vi "JsonFile Load.vi"(8 "error in (no error)":errorcluster, 11 "Path":path) -> (0 "error out":errorcluster, 3 "Json":string)   [LabVIEW 2019, in "lv-apt-json-file.lvlib"]
uses:
  lv-apt-json-file.lvlib
  <vilib>/JDP Science/JSONtext/JSONtext.lvlib
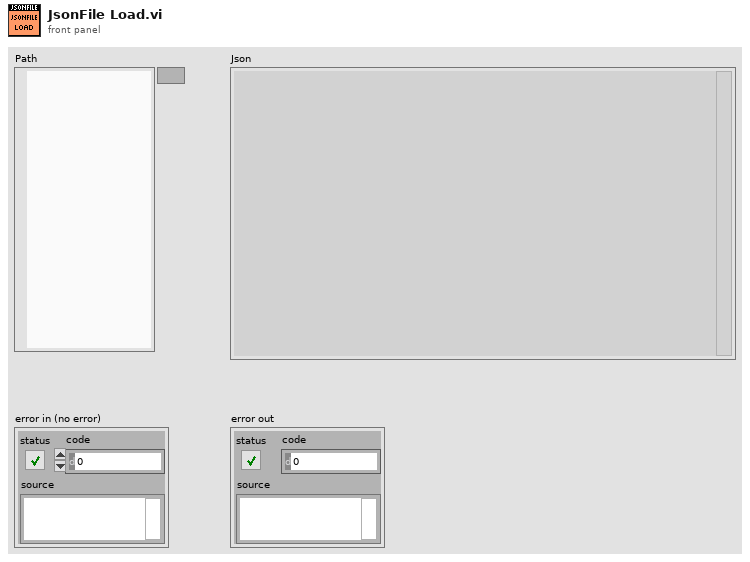
[diagram p1: front panel]
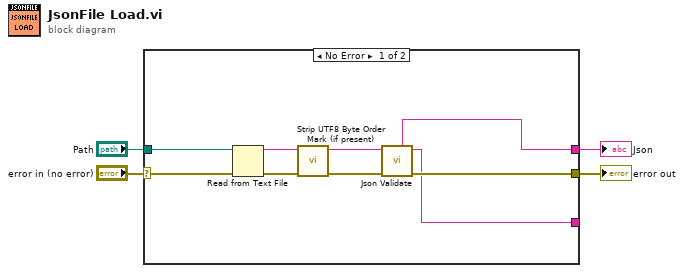
[diagram p0: block diagram]
diagram:
  n1 = case shown="No Error" "error in (no error)" {
    selector: "error in (no error)" -> [w5 w13]
    tunnel: "Path" -> [w8 _]
    tunnel: [w11 _] -> w2
    tunnel: [w12 w13] -> w1
    tunnel: [w10 _] -> _
    frame No Error {
      n2 = Read from Text File(file (use dialog)=w8, error in=w5) -> (text=w9:string, error out=w6:errorcluster)  [unwired: 2 in, 2 out]
      n3 = call <vilib>:"Strip UTF8 Byte Order Mark (if present).vi"("Text in"=w9) -> ("Possible Byte Order Mark Stripped"=w7:string)  [unwired: 9 in, 1 out]
      n4 = call "Json Validate.vi"("error in (no error)"=w6, "String"=w7) -> ("error out"=w12:errorcluster, "Json without comments"=w10:string, "String (dup)"=w11:string)  [unwired: 6 in, 1 out]
    }
    frame Error {
    }
  }
  "error out" <- w1
  "Json" <- w2
